vi "str2array.vi"(1 "string in":string) -> (0 "array out":dbl[](array[numeric]) format="%.2f")   [LabVIEW 2017]
doc: "Transforms a string of number delimted by spaces into an array."
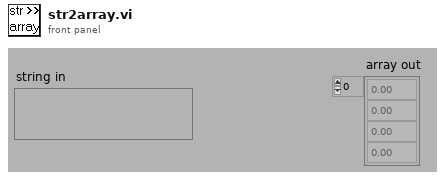
[diagram p1: front panel]
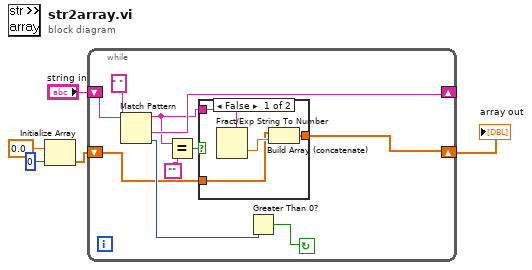
[diagram p0: block diagram]
diagram:
  n1 = Initialize Array(0.0, 0) -> (w1:dbl[])
  n2 = while {
    shift-left: w1 -> [w7]
    shift-right: [w6] -> w4
    shift-left: "string in" -> [w15]
    shift-right: [w14] -> _
    stop <- w12 continue-if-true
    n3 = Match Pattern(string=w15, regular expression=" ") -> (before substring=w10:string, after substring=w14:string, offset past match=w13:i32)  [unwired: 1 in, 1 out]
    n4 = Equal?(x=w10, y="") -> (x = y?=w8:bool)
    n5 = case shown="False" w8 {
      tunnel: w10 -> [w19 _]
      tunnel: w7 -> [w17 w20]
      tunnel: [w16 w20] -> w6
      frame False {
        n6 = Fract/Exp String To Number(string=w19) -> (number=w18:dbl)  [unwired: 3 in, 1 out]
        n7 = Build Array (concatenate)(w17, w18) -> (w16:dbl[])
      }
      frame True {
      }
    }
    n8 = Greater Than 0?(x=w13) -> (x > 0?=w12:bool)
  }
  "array out" <- w4
